vi "HandleItemActivation.vi"(8 "error in (no error)":errorcluster, 11 "Link in":refnum<class "Link.lvclass">) -> (0 "error out":errorcluster, 3 "Link out":refnum<class "Link.lvclass">)   [LabVIEW 2009, in "NavScreen.lvlib" / "Link.lvclass"]
uses:
  Link.lvclass
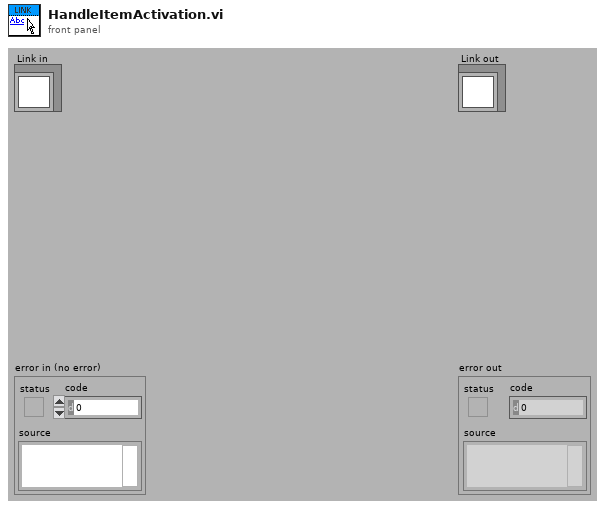
[diagram p1: front panel]
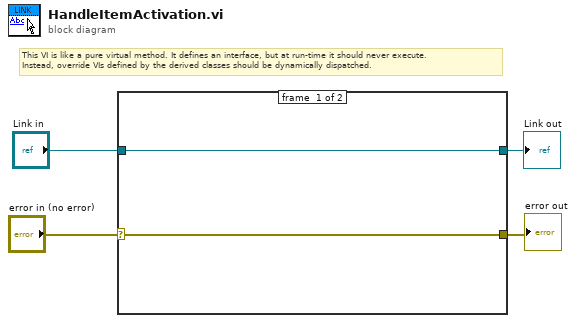
[diagram p0: block diagram]
diagram:
  # "This VI is like a pure virtual method. It defines an interface, but at run-time it should never execute.\nInstead, override VIs defined by the derived classes should be dynamically dispatched."
  n1 = case shown="No Error" "error in (no error)" {
    selector: "error in (no error)" -> [w5 w8]
    tunnel: [w5 w8] -> w3
    tunnel: [w6 w7] -> w1
    tunnel: "Link in" -> [w6 w7]
    frame #0 {
    }
    frame #1 {
    }
  }
  "error out" <- w3
  "Link out" <- w1
